vi "DCA Append Group Data Fields.vi"(10 "DCA Results":T1, 11 "Fields In":T12[](array[typedef])) -> (3 "Fields Out":T12[](array[typedef]))   [LabVIEW 2011]
uses:
  server/database/Fields/Field Record.ctl
  server/database/Fields/Field DataTypes.ctl
  server/database/Fields/Field NextItem.ctl
  TypeDefs/DCA Results.ctl
  TypeDefs/DCA Measurement Values.ctl
  TypeDefs/DCA Topology.ctl
  TypeDefs/DCA Limit.ctl
  TypeDefs/DCA Limit Quantity.ctl
  TypeDefs/DCA Limit Comparison.ctl
  TypeDefs/DCA Limit Operation.ctl
  Test Referential Limit.ctl
  TypeDefs/DCA Calibration State.ctl
  TypeDefs/DCA Attenuation Calculation.ctl
  server/database/Stations/Instruments/Instrument Record.ctl
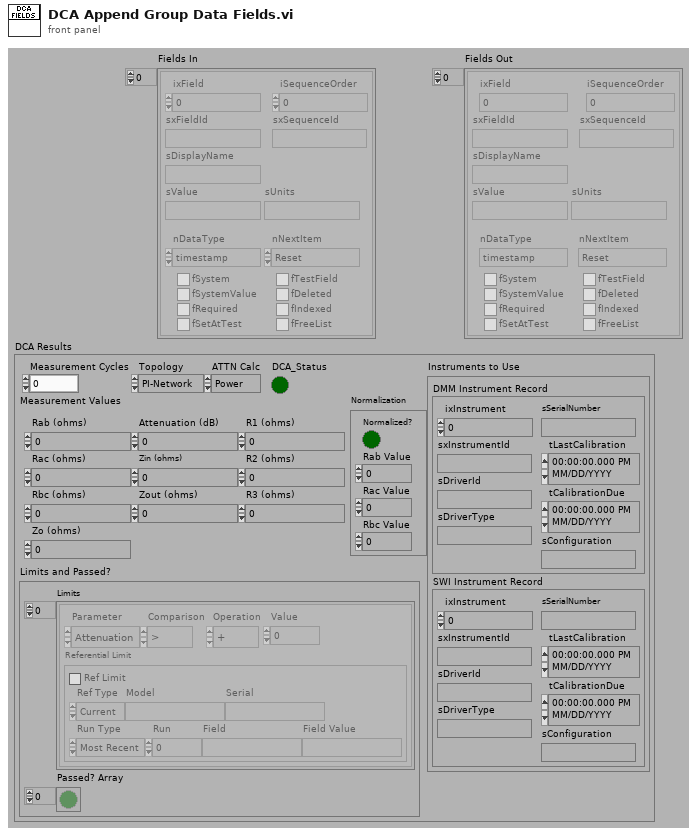
[diagram p1: front panel]
types:
  T1 = typedef "DCA Results.ctl" = cluster{"Measurement Cycles":i32, "Measurement Values":T2, "Topology":T3, "DCA_Status":bool, "Limits and Passed?":cluster{"Limits":T4[], "Passed? Array":bool[]}, "Normalization":T9, "ATTN Calc":T10, "Instruments to Use":cluster{"DMM Instrument Record":T11, "SWI Instrument Record":T11}}
  T2 = typedef "DCA Measurement Values.ctl" = cluster{"Rab (ohms)":dbl, "Rac (ohms)":dbl, "Rbc (ohms)":dbl, "Zo (ohms)":dbl, "Attenuation (dB)":dbl, "Zin (ohms)":dbl, "Zout (ohms)":dbl, "R1 (ohms)":dbl, "R2 (ohms)":dbl, "R3 (ohms)":dbl}
  T3 = typedef "DCA Topology.ctl" = enum32{"PI-Network", "T-Network"}
  T4 = typedef "DCA Limit.ctl" = cluster{"Parameter":T5, "Comparison":T6, "Operation":T7, "Value":dbl, "Referential Limit":T8}
  T5 = typedef "DCA Limit Quantity.ctl" = enum16{"Attenuation", "Zin", "Zout", "R1", "R2", "R3", "Rab", "Rac", "Rbc"}
  T6 = typedef "DCA Limit Comparison.ctl" = enum16{">", ">=", "<", "<="}
  T7 = typedef "DCA Limit Operation.ctl" = enum16{"+", "-"}
  T8 = typedef "Test Referential Limit.ctl" = cluster{"Ref Limit":bool, "Ref Type":enum16{"Current", "Specify"}, "Model":string, "Serial":string, "Run Type":enum16{"Most Recent", "Run #", "Match Field"}, "Run":i32, "Field":string, "Field Value":string}
  T9 = typedef "DCA Calibration State.ctl" = cluster{"Normalized?":bool, "Rab Value":dbl, "Rac Value":dbl, "Rbc Value":dbl}
  T10 = typedef "DCA Attenuation Calculation.ctl" = enum32{"Power", "Voltage"}
  T11 = typedef "Instrument Record.ctl" = cluster{"ixInstrument":i32, "sxInstrumentId":string, "sDriverId":string, "sDriverType":string, "sSerialNumber":string, "tLastCalibration":timestamp, "tCalibrationDue":timestamp, "sConfiguration":string}
  T12 = typedef "Field Record.ctl" = cluster{"ixField":i32, "iSequenceOrder":i32, "sxFieldId":string, "sxSequenceId":string, "sDisplayName":string, "sValue":string, "sUnits":string, "nDataType":T13, "nNextItem":T14, "fSystem":bool, "fSystemValue":bool, "fRequired":bool, "fSetAtTest":bool, "fTestField":bool, "fDeleted":bool, "fIndexed":bool, "fFreeList":bool}
  T13 = typedef "Field DataTypes.ctl" = enum32{"text", "numeric", "list", "timestamp", "boolean"}
  T14 = typedef "Field NextItem.ctl" = enum32{"Reset", "Retain", "Auto-Increment"}
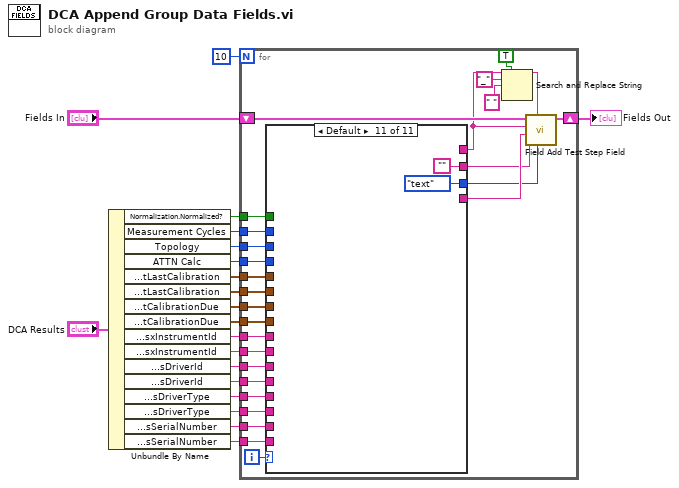
[diagram p0: block diagram]
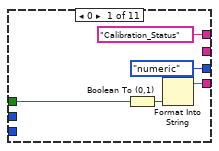
[diagram p2: hidden frame]
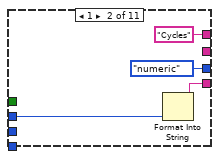
[diagram p3: hidden frame]
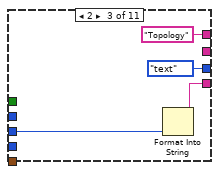
[diagram p4: hidden frame]
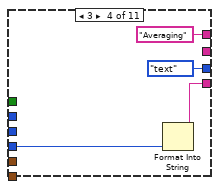
[diagram p5: hidden frame]
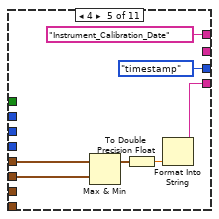
[diagram p6: hidden frame]
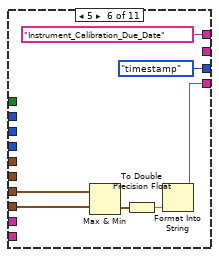
[diagram p7: hidden frame]
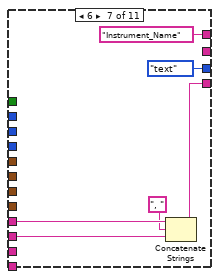
[diagram p8: hidden frame]
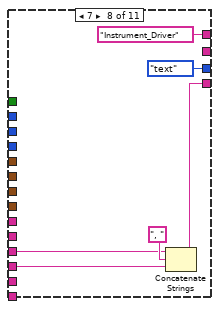
[diagram p9: hidden frame]
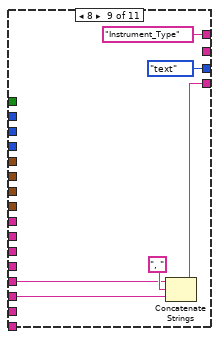
[diagram p10: hidden frame]
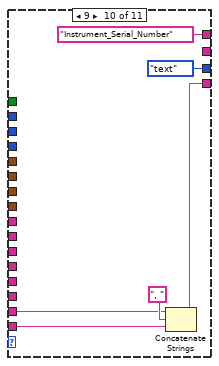
[diagram p11: hidden frame]
diagram:
  n1 = Unbundle By Name("DCA Results") -> ("Normalization.Normalized?"=w16:bool, "Measurement Cycles"=w15:i32, "Topology"=w14:T3, "ATTN Calc"=w13:T10, "Instruments to Use.DMM Instrument Record.tLastCalibration"=w12:timestamp, "Instruments to Use.SWI Instrument Record.tLastCalibration"=w11:timestamp, "Instruments to Use.DMM Instrument Record.tCalibrationDue"=w10:timestamp, "Instruments to Use.SWI Instrument Record.tCalibrationDue"=w9:timestamp, "Instruments to Use.DMM Instrument Record.sxInstrumentId"=w8:string, "Instruments to Use.SWI Instrument Record.sxInstrumentId"=w7:string, "Instruments to Use.DMM Instrument Record.sDriverId"=w6:string, "Instruments to Use.SWI Instrument Record.sDriverId"=w5:string, "Instruments to Use.DMM Instrument Record.sDriverType"=w4:string, "Instruments to Use.SWI Instrument Record.sDriverType"=w3:string, "Instruments to Use.DMM Instrument Record.sSerialNumber"=w2:string, "Instruments to Use.SWI Instrument Record.sSerialNumber"=w1:string)
  n2 = for {
    N: 10 -> [_]
    tunnel: w13 -> [w46]
    tunnel: w14 -> [w45]
    tunnel: w15 -> [w44]
    tunnel: w16 -> [w43]
    shift-right: [w41] -> w19
    shift-left: "Fields In" -> [w42]
    tunnel: w12 -> [w37]
    tunnel: w11 -> [w36]
    tunnel: w10 -> [w35]
    tunnel: w9 -> [w34]
    tunnel: w8 -> [w33]
    tunnel: w7 -> [w32]
    tunnel: w6 -> [w31]
    tunnel: w5 -> [w30]
    tunnel: w4 -> [w29]
    tunnel: w3 -> [w28]
    tunnel: w2 -> [w27]
    tunnel: w1 -> [w26]
    i -> [w47]
    n3 = case shown="Default" w47 {
      tunnel: w46 -> [_ _ _ w61 _ _ _ _ _ _ _]
      tunnel: w45 -> [_ _ w58 _ _ _ _ _ _ _ _]
      tunnel: w44 -> [_ w54 _ _ _ _ _ _ _ _ _]
      tunnel: w43 -> [w49 _ _ _ _ _ _ _ _ _ _]
      tunnel: ["Calibration_Status" ("Field_ID") "Cycles" ("Field_ID") "Topology" ("Field_ID") "Averaging" ("Field_ID") "Instrument_Calibration_Date" ("Field_ID") "Instrument_Calibration_Due_Date" ("Field_ID") "Instrument_Name" ("Field_ID") "Instrument_Driver" ("Field_ID") "Instrument_Type" ("Field_ID") "Instrument_Serial_Number" ("Field_ID") _] -> w22
      tunnel: [Field_DataTypes."numeric" ("Data Type") Field_DataTypes."numeric" ("Data Type") Field_DataTypes."text" ("Data Type") Field_DataTypes."text" ("Data Type") Field_DataTypes."timestamp" ("Data Type") Field_DataTypes."timestamp" ("Data Type") Field_DataTypes."text" ("Data Type") Field_DataTypes."text" ("Data Type") Field_DataTypes."text" ("Data Type") Field_DataTypes."text" ("Data Type") Field_DataTypes."text" ("Data Type")] -> w39
      tunnel: [w51 w55 w57 w62 w68 w75 w81 w88 w94 w100 _] -> w40
      tunnel: [_ _ _ _ _ _ _ _ _ _ ""] -> w38
      tunnel: w37 -> [_ _ _ _ w67 _ _ _ _ _ _]
      tunnel: w36 -> [_ _ _ _ w66 _ _ _ _ _ _]
      tunnel: w35 -> [_ _ _ _ _ w74 _ _ _ _ _]
      tunnel: w34 -> [_ _ _ _ _ w73 _ _ _ _ _]
      tunnel: w33 -> [_ _ _ _ _ _ w82 _ _ _ _]
      tunnel: w32 -> [_ _ _ _ _ _ w80 _ _ _ _]
      tunnel: w31 -> [_ _ _ _ _ _ _ w86 _ _ _]
      tunnel: w30 -> [_ _ _ _ _ _ _ w85 _ _ _]
      tunnel: w29 -> [_ _ _ _ _ _ _ _ w92 _ _]
      tunnel: w28 -> [_ _ _ _ _ _ _ _ w91 _ _]
      tunnel: w27 -> [_ _ _ _ _ _ _ _ _ w98 _]
      tunnel: w26 -> [_ _ _ _ _ _ _ _ _ w97 _]
      frame 0 {
        n4 = Boolean To (0,1)(Boolean=w49) -> (0, 1=w48:i16)
        n5 = Format Into String(w48) -> (resulting string=w51:string)  [unwired: 3 in, 1 out]
      }
      frame 1 {
        n6 = Format Into String(w54) -> (resulting string=w55:string)  [unwired: 3 in, 1 out]
      }
      frame 2 {
        n7 = Format Into String(w58) -> (resulting string=w57:string)  [unwired: 3 in, 1 out]
      }
      frame 3 {
        n8 = Format Into String(w61) -> (resulting string=w62:string)  [unwired: 3 in, 1 out]
      }
      frame 4 {
        n9 = Max & Min(x=w67, y=w66) -> (max(x,y)=w65:timestamp)  [unwired: 1 out]
        n10 = To Double Precision Float(number=w65) -> (double precision float=w69:dbl)
        n11 = Format Into String(w69) -> (resulting string=w68:string)  [unwired: 3 in, 1 out]
      }
      frame 5 {
        n12 = Max & Min(x=w74, y=w73) -> (min(x,y)=w72:timestamp)  [unwired: 1 out]
        n13 = To Double Precision Float(number=w72) -> (double precision float=w76:dbl)
        n14 = Format Into String(w76) -> (resulting string=w75:string)  [unwired: 3 in, 1 out]
      }
      frame 6 {
        n15 = Concatenate Strings(w82, ", ", w80) -> (w81:string)
      }
      frame 7 {
        n16 = Concatenate Strings(w86, ", ", w85) -> (w88:string)
      }
      frame 8 {
        n17 = Concatenate Strings(w92, ", ", w91) -> (w94:string)
      }
      frame 9 {
        n18 = Concatenate Strings(w98, ", ", w97) -> (w100:string)
      }
      frame Default {
      }
    }
    n19 = Search and Replace String(replace all?=TRUE ("replace all? (F)"), input string=w22, search string="_", replace string=" " ("replace string (\"\")")) -> (result string=w21:string)  [unwired: 1 in, 6 out]
    n20 = call "Field Add Test Step Field.vi"("nDataType"=w39, "sDisplayName"=w21, "sUnits"=w38, "sValue"=w40, "sxFieldId"=w22, "Fields In"=w42) -> ("Fields Out"=w41:T12[])  [unwired: 5 out]
  }
  "Fields Out" <- w19
